vi "ARRAY2DHandle.vi"() -> ()   [LabVIEW 2023]
doc: "This function squares each value in the 2-D array.\n\nFor information on the data types used for the DLL function, right-click on the Call Library Function node and choose Configure."
uses:
  CLF_Example.dll
panel:
  out "output":dbl[][](array[numeric])
  in  "input":dbl[][](array[numeric])=[[0.0, 1.0], [2.0, 3.0], [4.0, 5.0], [6.0, 7.0]]
  # "See the block diagram for more information."
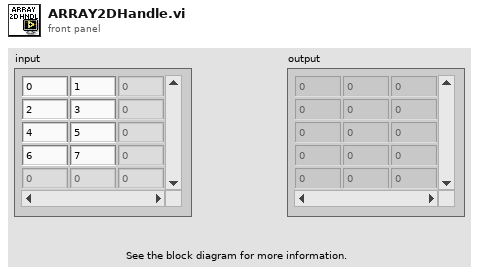
[diagram p1: front panel]
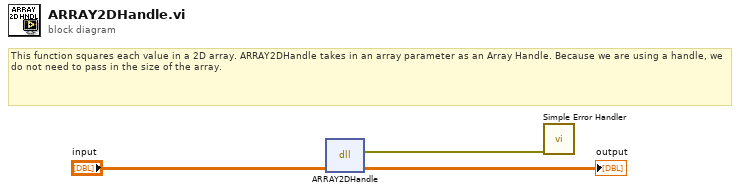
[diagram p0: block diagram]
diagram:
  # "This function squares each value in a 2D array. ARRAY2DHandle takes in an array parameter as an Array Handle. Because we are using a handle, we do not need to pass in the size of the array."
  n1 = dll-call lib="c:/dev/_r/4/eng/lv-core/lvpostprocessingd/lv_mc_x86_64/dist_i386/examples/Connectivity/Libraries and Executables/DLL Calling VIs/CLF_Example**.*" fn="ARRAY2DHandle"("array"="input") -> (error out=w1:errorcluster, "array"=→"output":dbl[][])  [unwired: 3 in, 2 out]
  n2 = call <vilib>:"Simple Error Handler.vi"("error in (no error)"=w1) -> ()  [unwired: 4 in, 5 out]
